vi "Main.vi"(8 "error in (no error)":errorcluster, 10 "MODO":T2=enum."CONFIG ESTACION", 11 "VISA sesion":refnum<visa-resource-name>) -> (0 "error out":errorcluster, 3 "VISA resource name":refnum<visa-resource-name>)   [LabVIEW 2019]
doc: "Use this template to build a simple state machine design pattern. Each state executes code and determines which state to transition to."
uses:
  Type_defs/Coordenadas_estacion.ctl
  LABVIEW_ROBOT_MASTER/Type_defs/TAREAS_ROBOT.ctl
  Type_defs/state_config_estacion.ctl
  <vilib>/Utility/xml.llb/Write to XML File(string).vi
  SHARED VI'S/SHARED VI'S.lvlib
panel:
  in  "Tab Control":enum32{"Page 1", "Page 2"}(tab)
  in  "EXIT":bool
  out "Ruta y fichero de configuración de bandeja seleccionado":path
  in  "Crear/Seleccionar bandeja":bool caption="Crear bandeja"
  out "Ruta y fichero de configuración estación":path
  in  "Tab depuracion":enum32{"Page 1", "Page 2"}(tab)
  out "Coordenadas_estacion":T1
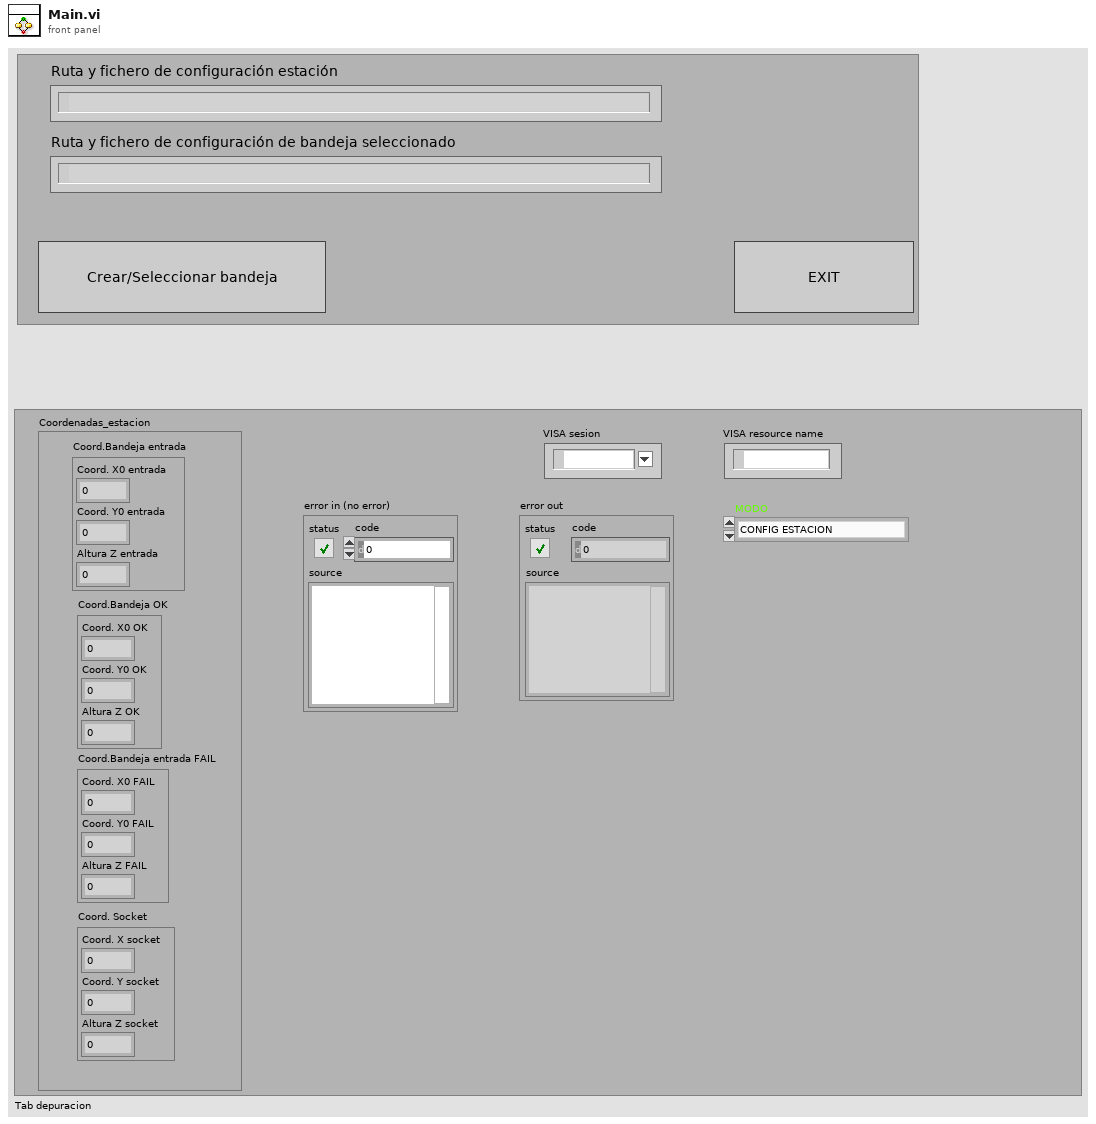
[diagram p1: front panel]
types:
  T1 = typedef "Coordenadas_estacion.ctl" = cluster{"Coord.Bandeja entrada":cluster{"Coord. X0 entrada":u32, "Coord. Y0 entrada ":u32, "Altura Z entrada":u32}, "Coord.Bandeja OK":cluster{"Coord. X0 OK":u32, "Coord. Y0 OK":u32, "Altura Z OK":u32}, "Coord.Bandeja entrada FAIL":cluster{"Coord. X0 FAIL":u32, "Coord. Y0 FAIL":u32, "Altura Z FAIL":u32}, "Coord. Socket":cluster{"Coord. X socket":u32, "Coord. Y socket":u32, "Altura Z socket":u32}}
  T2 = typedef "TAREAS_ROBOT.ctl" = enum16{"NINGUNA", "TEST ASICS", "AJUSTE CAM", "MOVER ASICS", "MOVIMIENTO MANUAL", "LEER QR", "CONFIG ESTACION"}
  T3 = typedef "state_config_estacion.ctl" = enum16{"Init", "Get coordenadas", "Crear bandeja JEDEC", "Guardar config estacion", "Evento", "Exit", "Error"}
  T4 = enum8{"Enabled", "Disabled", "Disabled and Grayed Out"}
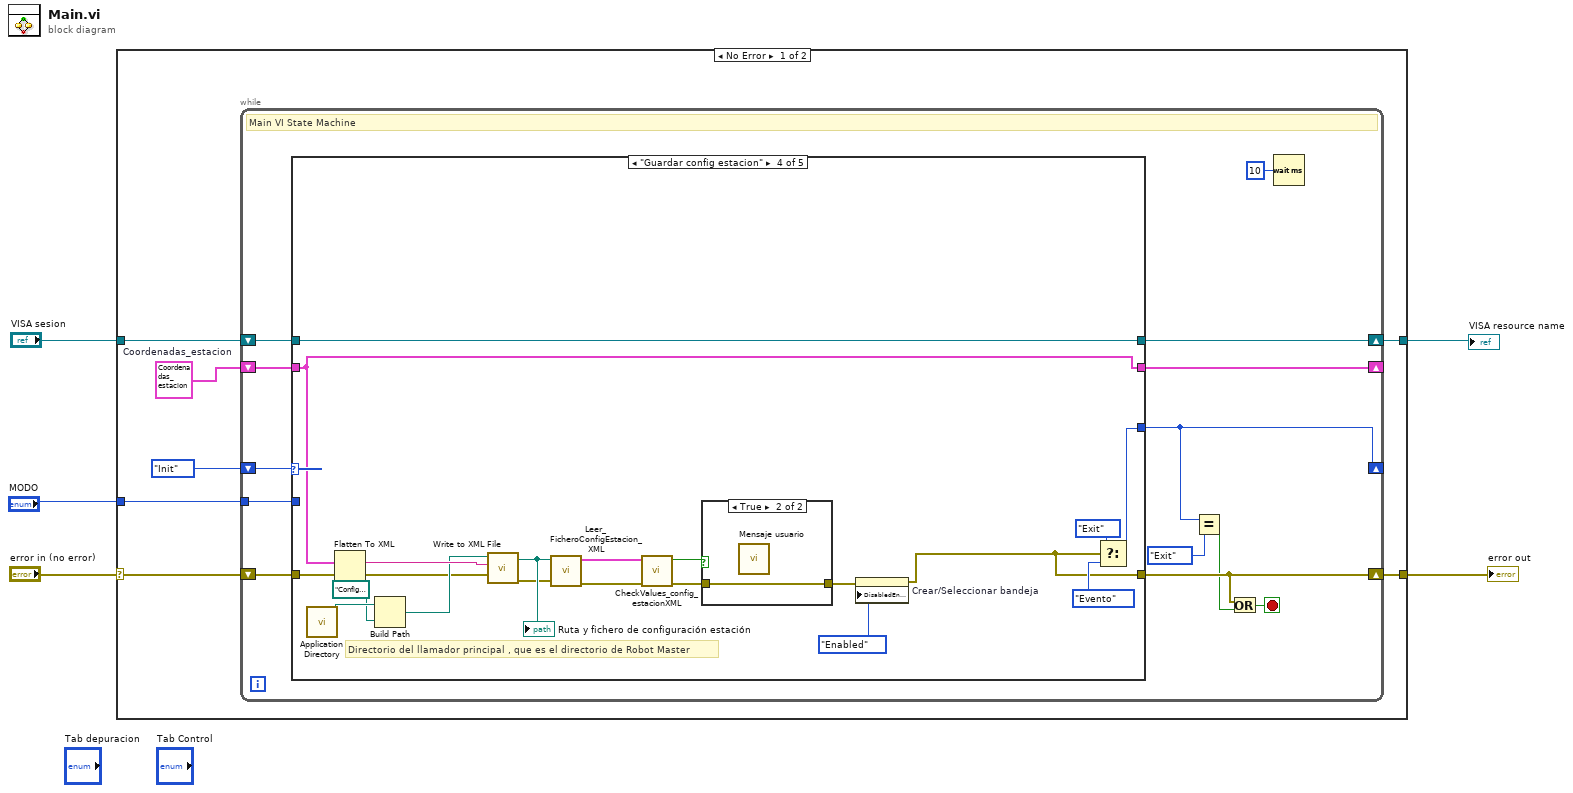
[diagram p0: block diagram]
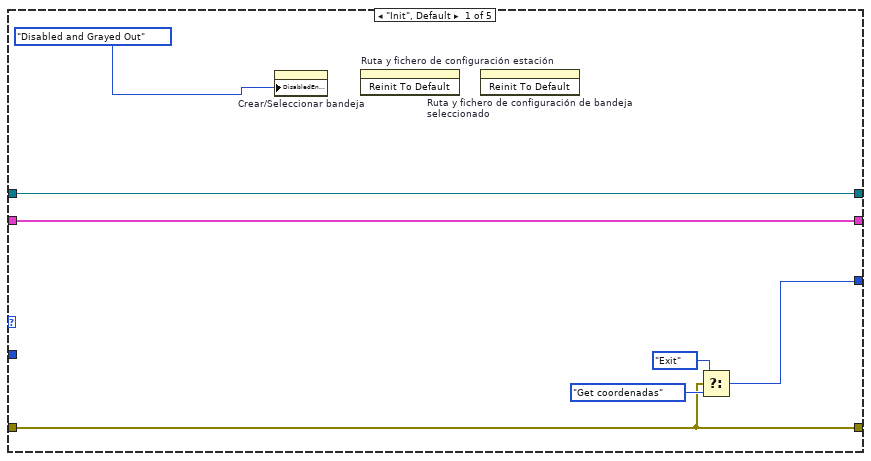
[diagram p2: hidden frame]
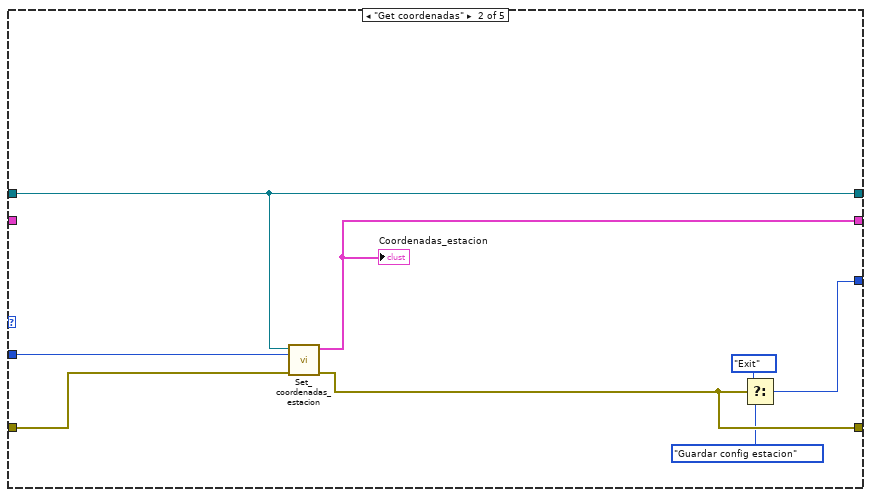
[diagram p3: hidden frame]
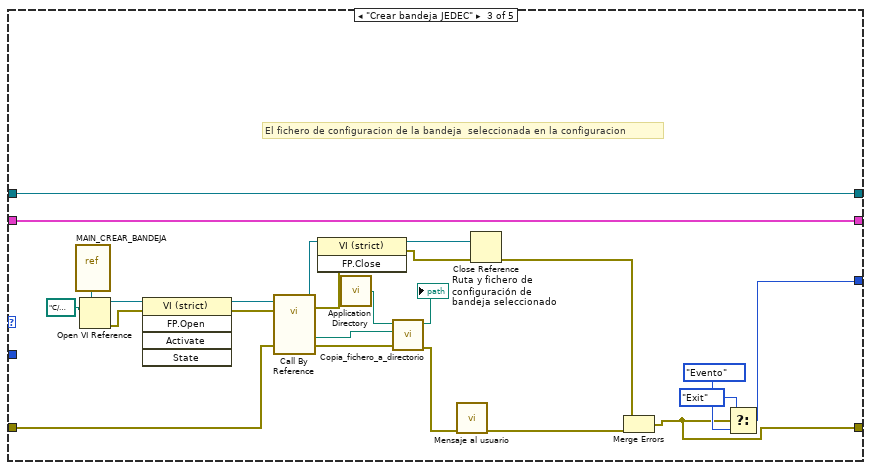
[diagram p4: hidden frame]
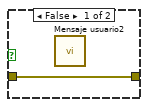
[diagram p5: hidden frame]
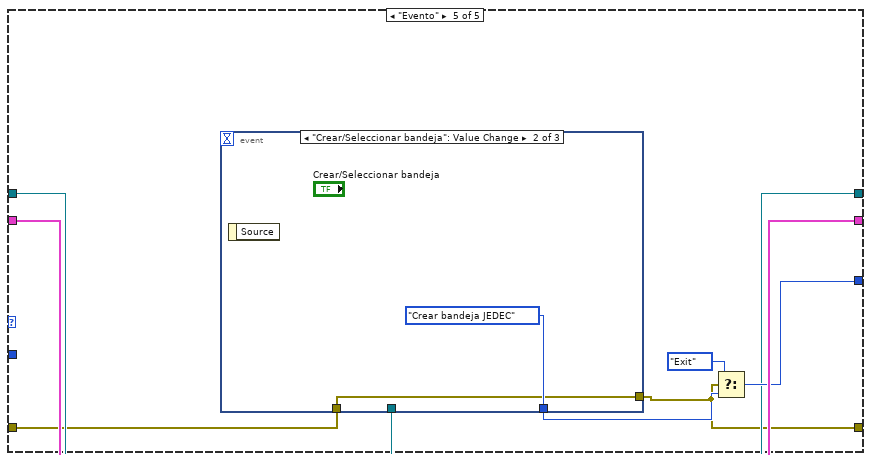
[diagram p6: hidden frame]
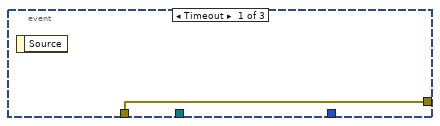
[diagram p7: hidden frame]
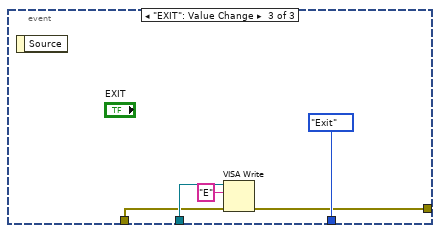
[diagram p8: hidden frame]
diagram:
  n1 = case shown="No Error" "error in (no error)" {
    selector: "error in (no error)" -> [w11 w101]
    tunnel: [w12 w101] -> w5
    tunnel: "VISA sesion" -> [w10 w102]
    tunnel: [w9 w102] -> w2
    tunnel: "MODO" -> [w6 _]
    frame No Error {
      w8 = T1 {"Coord.Bandeja entrada"={"Coord. X0 entrada"=0, "Coord. Y0 entrada "=0, "Altura Z entrada"=0}, "Coord.Bandeja OK"={"Coord. X0 OK"=0, "Coord. Y0 OK"=0, "Altura Z OK"=0}, "Coord.Bandeja entrada FAIL"={"Coord. X0 FAIL"=0, "Coord. Y0 FAIL"=0, "Altura Z FAIL"=0}, "Coord. Socket"={"Coord. X socket"=0, "Coord. Y socket"=0, "Altura Z socket"=0}}  # Coordenadas_estacion
      n2 = while {
        shift-right: [w23] -> w12
        shift-left: w11 -> [w25]
        shift-right: [w19] -> w9
        shift-left: w10 -> [w20]
        shift-right: [w18] -> _
        shift-left: w8 -> [w17]
        shift-right: [w15] -> _
        shift-left: state_config_estacion."Init" ("Estado") -> [w16]
        tunnel: w6 -> [w13]
        stop <- w24 stop-if-true
        # "Main VI State Machine"
        n3 = case shown="\"Guardar config estacion\"" w16 {
          tunnel: w25 -> [w30 w39 w56 w79 w87]
          tunnel: [w30 w38 w48 w65 w86] -> w23
          tunnel: w20 -> [w29 w37 w63 w83 w88]
          tunnel: [w29 w37 w63 w83 w88] -> w19
          tunnel: [w28 w36 w64 w74 w90] -> w18
          tunnel: w17 -> [w28 _ w64 w74 w90]
          tunnel: [w27 w34 w47 w76 w89] -> w15
          tunnel: w13 -> [_ w33 _ _ _]
          frame "Init", Default {
            # "Initialize - Initialize the application."
            n4 = property on="Crear/Seleccionar bandeja" class="Bool"("DisabledEnum"=T4."Disabled and Grayed Out" ("Disabled")) -> ()  [unwired: 2 in, 2 out]
            n5 = invoke on="Ruta y fichero de configuración estación" class="Path" method="Reinit To Default"() -> ()  [unwired: 3 in, 3 out]
            n6 = invoke on="Ruta y fichero de configuración de bandeja seleccionado" class="Path" method="Reinit To Default"() -> ()  [unwired: 3 in, 3 out]
            n7 = Select(t=state_config_estacion."Exit" ("Estado"), s=w30, f=state_config_estacion."Get coordenadas") -> (s? t:f=w27:T3)
          }
          frame "Get coordenadas" {
            # "Wait for Event - Use an Event Structure to monitor the user interface for events that run different states of the state machine."
            n8 = call "Set_coordenadas_estacion.vi"("error in (no error)"=w39, "MODO"=w33, "VISA SESSION"=w37) -> ("error out"=w38:errorcluster, "Coordenadas_estacion 2"=w36:T1)  [unwired: 7 in]
            "Coordenadas_estacion" <- w36
            n9 = Select(t=state_config_estacion."Exit" ("Estado"), s=w38, f=state_config_estacion."Guardar config estacion") -> (s? t:f=w34:T3)
          }
          frame "Crear bandeja JEDEC" {
            # "El fichero de configuracion de la bandeja  seleccionada en la configuracion"
            # "User State 1 - Replace this state with functionality for your own application."
            n10 = vi-ref "MAIN_CREAR_BANDEJA.vi"() -> (w62:refnum<vi>)
            n11 = Open VI Reference(type specifier VI Refnum (for type only)=w62, vi path=path "C:/Trabajo_Robot/TFG_ROBOT/CONTROL_ROBOT/LVPROJ_CREAR BANDEJAS/MAIN_CREAR_BANDEJA.vi") -> (vi reference=w60:refnum<vi>, error out=w55:errorcluster)  [unwired: 4 in]
            n12 = invoke class="VI (strict)" method="FP.Open"(reference=w60, error in=w55) -> (reference out=w59:refnum<vi>, error out=w54:errorcluster)  [unwired: 3 in, 3 out]
            n13 = call-by-ref "?"(reference=w59, error in=w54, 8:"error in (no error)"=w56) -> (reference out=w58:refnum<vi>, error out=w53:errorcluster, "error in (no error) 2"=w44:errorcluster, "fichero bandeja selecc"=w45:path)  [unwired: 9 in]
            n14 = invoke class="VI (strict)" method="FP.Close"(reference=w58, error in=w53) -> (reference out=w57:refnum<vi>, error out=w52:errorcluster)  [unwired: 1 in, 1 out]
            n15 = call <vilib>:"Application Directory.vi"() -> ("Application Directory"=w46:path)
            n16 = call "Copia_fichero_a_directorio.vi"("error in (no error)"=w44, "source path"=w45, "Target path"=w46) -> ("error out"=w42:errorcluster, "new path"=→"Ruta y fichero de configuración de bandeja seleccionado":path)  [unwired: 7 in]
            n17 = call "Mensaje al usuario"("error in (no error)"=w42) -> ("error out"=w41:errorcluster)  [unwired: 9 in, 1 out]
            n18 = Close Reference(reference=w57, error in (no error)=w52) -> (error out=w51:errorcluster)
            n19 = Merge Errors(w51, w41) -> (w48:errorcluster)
            n20 = Select(t=state_config_estacion."Exit" ("Estado"), s=w48, f=state_config_estacion."Evento") -> (s? t:f=w47:T3)
          }
          frame "Guardar config estacion" {
            # "Directorio del llamador principal , que es el directorio de Robot Master"
            # "User State 2 - Replace this state with functionality for your own application."
            n21 = call <vilib>:"Application Directory.vi"() -> ("Application Directory"=w82:path)
            n22 = Flatten To XML(anything=w74) -> (xml string=w81:string)
            n23 = Build Path(base path=w82, name or relative path=path "Config_file_estacion.xml") -> (appended path=w80:path)
            n24 = call-poly <vilib>:"Write to XML File.vi"("error in (no error)"=w79, "XML Input"=w81, "XML File Path"=w80) -> ("error out"=w71:errorcluster, "XML File Path(duplicate)"=w72:path)  [unwired: 6 in, 1 out]
            "Ruta y fichero de configuración estación" <- w72
            n25 = call "Leer_FicheroConfigEstacion_XML.vi"("error in (no error)"=w71, "XML File Path"=w72) -> ("error out"=w69:errorcluster, "Coordenadas_estacion"=w70:T1)  [unwired: 8 in]
            n26 = call "CheckValues_config_estacionXML.vi"("error in (no error)"=w69, "Coordenadas_estacion"=w70) -> ("error out"=w68:errorcluster, "XML NULL?"=w66:bool)  [unwired: 8 in]
            n27 = case shown="True" w66 {
              tunnel: w68 -> [w84 w85]
              tunnel: [w84 w85] -> w67
              frame False {
                n28 = call "Mensaje usuario2"() -> ()  [unwired: 10 in, 2 out]
              }
              frame True {
                n29 = call "Mensaje usuario"() -> ()  [unwired: 10 in, 2 out]
              }
            }
            n30 = property on="Crear/Seleccionar bandeja" class="Bool"(error in=w67, "DisabledEnum"=T4."Enabled" ("Disabled")) -> (error out=w65:errorcluster)  [unwired: 1 in, 1 out]
            n31 = Select(t=state_config_estacion."Exit" ("Estado"), s=w65, f=state_config_estacion."Evento") -> (s? t:f=w76:T3)
          }
          frame "Evento" {
            n32 = event shown="[1] \"Crear/Seleccionar bandeja\": Value Change" {
              selector: _ -> [_ _ _]
              dyn-events: _ -> [_ _ _]
              timeout: _ -> [_ _ _]
              tunnel: [_ state_config_estacion."Crear bandeja JEDEC" ("f") state_config_estacion."Exit" ("f")] -> w91
              tunnel: w88 -> [_ _ w99]
              tunnel: w87 -> [w93 w94 w97]
              tunnel: [w93 w94 w96] -> w86
              event Timeout {
                n33 = event-data() -> ()  [unwired: 1 in, 1 out]
              }
              event "Crear/Seleccionar bandeja": Value Change {
                n34 = event-data() -> ()  [unwired: 1 in, 1 out]
              }
              event "EXIT": Value Change {
                n35 = event-data() -> ()  [unwired: 1 in, 1 out]
                n36 = VISA Write(VISA resource name=w99, write buffer="E", error in (no error)=w97) -> (error out=w96:errorcluster)  [unwired: 2 out]
              }
            }
            n37 = Select(t=state_config_estacion."Exit" ("Estado"), s=w86, f=w91) -> (s? t:f=w89:T3)
          }
        }
        n38 = Equal?(x=w15, y=state_config_estacion."Exit" ("Estado")) -> (x = y?=w21:bool)
        n39 = Or(x=w23, y=w21) -> (x .or. y?=w24:bool)
        n40 = Wait (ms)(milliseconds to wait=u32 10) -> ()  [unwired: 1 out]
      }
    }
    frame Error {
    }
  }
  "error out" <- w5
  "VISA resource name" <- w2
